vi "UHR-Fleezers Control (host) - Lorentz v2.vi"() -> ()   [LabVIEW 2014] (continued)
                            tunnel: [w3947] -> w3939
                            tunnel: [w3946] -> w3938
                            tunnel: w3937 -> [w3945]
                            tunnel: [w3945] -> w3936
                            tunnel: w3935 -> [w3944]
                            tunnel: [w3944] -> w3934
                            tunnel: [w4020] -> w3942
                            tunnel: w3940 -> [w4020]
                            tunnel: w3939 -> [w4019]
                            tunnel: w3938 -> [w4018]
                            tunnel: w3936 -> [w4017]
                            tunnel: w3934 -> [w4016]
                            frame #0 {
                              n2583 = call <vilib>:"Beep.vi"() -> ()  [unwired: 12 in]
                              n2584 = local write "Waiting"(FALSE ("Waiting")) -> ()
                              n2585 = Increment(x=w3949) -> (x+1=w3948:i32)
                              n2586 = case shown="\"Image\"" w3946 {
                                tunnel: w3948 -> [_ w3954 _]
                                frame "Alarm", Default {
                                }
                                frame "Yank" {
                                n2587 = flat-sequence {
                                tunnel: w3954 -> [w3957]
                                tunnel: [w3956] -> w3953
                                tunnel: [w3955] -> w3952
                                tunnel: w3953 -> [w3967]
                                tunnel: w3952 -> [w3968]
                                frame #0 {
                                n2588 = local read "Yank Delay (s)"() -> (w3960:dbl)
                                n2589 = local read "N Array El"() -> (w3955:u8)
                                n2590 = Quotient & Remainder(x=w3957, y=w3955) -> (x-y*floor(x/y)=w3956:i32)  [unwired: 1 out]
                                n2591 = Multiply(x=w3960, y=1000.0) -> (x*y=w3958:dbl)
                                n2592 = Wait (ms)(milliseconds to wait=w3958) -> ()  [unwired: 1 out]
                                }
                                frame #1 {
                                n2593 = local read "Yank to which?"() -> (w3962:bool)
                                n2594 = local read "Random Choice"() -> (w3972:bool)
                                n2595 = local read "Yank to Trap Delta (MHz)"() -> (w3965:dbl[])
                                n2596 = local read "Yank to SP"() -> (w3966:dbl[])
                                n2597 = Random Number (0-1)() -> (number: 0 to 1=w3971:dbl)
                                n2598 = Multiply(x=w3968, y=w3971) -> (x*y=w3970:dbl)
                                n2599 = Round Toward -Infinity(1:w3970) -> (0:w3969:dbl)
                                n2600 = Select(t=w3969, s=w3972, f=w3967) -> (s? t:f=w3963:dbl)
                                n2601 = Select(t=w3965, s=w3962, f=w3966) -> (s? t:f=w3964:dbl[])
                                n2602 = Index Array(array=w3964, index=w3963) -> (element=w3961:dbl)
                                n2603 = case shown="True" w3962 {
                                tunnel: w3961 -> [w3973 w4000]
                                frame False {
                                n2604 = flat-sequence {
                                tunnel: w3973 -> [w3974]
                                frame #0 {
                                n2605 = property on="Trap Pos FB SP" class="DigNum (strict)"("Val(Sgnl)"=w3974) -> ()  [unwired: 2 in, 2 out]
                                }
                                frame #1 {
                                n2606 = Wait (ms)(milliseconds to wait=u32 700) -> ()  [unwired: 1 out]
                                }
                                frame #2 {
                                n2607 = local read "Action (%)"() -> (w3979:dbl)
                                n2608 = Absolute Value(x=w3979) -> (abs(x)=w3978:dbl)
                                n2609 = Greater?(x=w3978, y=70.0) -> (0:w3976:bool)
                                n2610 = property on="Remove Action Offset" class="Bool (strict)"("Val(Sgnl)"=w3976) -> ()  [unwired: 2 in, 2 out]
                                }
                                frame #3 {
                                n2611 = for {
                                N: 4 -> [_]
                                n2612 = flat-sequence {
                                frame #0 {
                                n2613 = Wait (ms)(milliseconds to wait=u32 500) -> ()  [unwired: 1 out]
                                }
                                frame #1 {
                                n2614 = local read "Action (%)"() -> (w3985:dbl)
                                n2615 = Absolute Value(x=w3985) -> (abs(x)=w3984:dbl)
                                n2616 = Greater?(x=w3984, y=70.0) -> (0:w3982:bool)
                                n2617 = property on="Remove Action Offset" class="Bool (strict)"("Val(Sgnl)"=w3982) -> ()  [unwired: 2 in, 2 out]
                                }
                                }
                                }
                                }
                                frame #4 {
                                n2618 = Wait (ms)(milliseconds to wait=u32 500) -> ()  [unwired: 1 out]
                                }
                                frame #5 {
                                n2619 = local read "Mean"() -> (w3993:dbl)
                                n2620 = Greater?(x=w3993, y=11.0) -> (0:w3987:bool)
                                n2621 = Not(x=w3987) -> (.not. x?=w3988:bool)
                                n2622 = And(x=w3988, y="Shift confocal") -> (x .and. y?=w3990:bool)
                                n2623 = And(x=w3987, y="Shift confocal") -> (x .and. y?=w3991:bool)
                                n2624 = case shown="True" w3991 {
                                frame False {
                                }
                                frame True {
                                n2625 = local read "Confocal Y 2 (V)"() -> (w3997:dbl)
                                n2626 = local read "Confocal X 2 (V)"() -> (w3996:dbl)
                                n2627 = property on="AO1" class="Slide (strict)"("Val(Sgnl)"=w3997) -> ()  [unwired: 2 in, 2 out]
                                n2628 = property on="AO2" class="Slide (strict)"("Val(Sgnl)"=w3996) -> ()  [unwired: 2 in, 2 out]
                                }
                                }
                                n2629 = case shown="True" w3990 {
                                frame False {
                                }
                                frame True {
                                n2630 = local read "Confocal Y 1 (V)"() -> (w3995:dbl)
                                n2631 = local read "Confocal X 1 (V)"() -> (w3994:dbl)
                                n2632 = property on="AO1" class="Slide (strict)"("Val(Sgnl)"=w3995) -> ()  [unwired: 2 in, 2 out]
                                n2633 = property on="AO2" class="Slide (strict)"("Val(Sgnl)"=w3994) -> ()  [unwired: 2 in, 2 out]
                                }
                                }
                                }
                                frame #6 {
                                n2634 = Wait (ms)(milliseconds to wait=u32 1500) -> ()  [unwired: 1 out]
                                }
                                frame #7 {
                                n2635 = property on="Rem fb disp offset" class="Bool (strict)"("Val(Sgnl)"=TRUE ("Value (Signaling)")) -> ()  [unwired: 2 in, 2 out]
                                }
                                }
                                }
                                frame True {
                                n2636 = flat-sequence {
                                tunnel: w4000 -> [w4001]
                                frame #0 {
                                n2637 = property on="Trap Delta (MHz)" class="DigNum (strict)"("Val(Sgnl)"=w4001) -> ()  [unwired: 2 in, 2 out]
                                }
                                frame #1 {
                                n2638 = Wait (ms)(milliseconds to wait=u32 500) -> ()  [unwired: 1 out]
                                }
                                frame #2 {
                                n2639 = local read "Shift confocal"() -> (w4007:bool)
                                n2640 = local read "Mean"() -> (w4009:dbl)
                                n2641 = Greater?(x=w4009, y=11.0) -> (0:w4006:bool)
                                n2642 = Not(x=w4006) -> (.not. x?=w4005:bool)
                                n2643 = And(x=w4005, y=w4007) -> (x .and. y?=w4003:bool)
                                n2644 = And(x=w4006, y=w4007) -> (x .and. y?=w4004:bool)
                                n2645 = case shown="True" w4004 {
                                frame False {
                                }
                                frame True {
                                n2646 = local read "Confocal Y 2 (V)"() -> (w4013:dbl)
                                n2647 = local read "Confocal X 2 (V)"() -> (w4012:dbl)
                                n2648 = property on="AO2" class="Slide (strict)"("Val(Sgnl)"=w4012) -> ()  [unwired: 2 in, 2 out]
                                n2649 = property on="AO1" class="Slide (strict)"("Val(Sgnl)"=w4013) -> ()  [unwired: 2 in, 2 out]
                                }
                                }
                                n2650 = case shown="True" w4003 {
                                frame False {
                                }
                                frame True {
                                n2651 = local read "Confocal X 1 (V)"() -> (w4010:dbl)
                                n2652 = local read "Confocal Y 1 (V)"() -> (w4011:dbl)
                                n2653 = property on="AO2" class="Slide (strict)"("Val(Sgnl)"=w4010) -> ()  [unwired: 2 in, 2 out]
                                n2654 = property on="AO1" class="Slide (strict)"("Val(Sgnl)"=w4011) -> ()  [unwired: 2 in, 2 out]
                                }
                                }
                                }
                                }
                                }
                                }
                                }
                                }
                                }
                                frame "Image" {
                                n2655 = property on="Confocal Image" class="Bool (strict)"("Val(Sgnl)"=TRUE ("Value (Signaling)")) -> ()  [unwired: 2 in, 2 out]
                                }
                              }
                              n2656 = local write "Fl. High"(FALSE ("Fl. High")) -> ()
                              n2657 = local read "Time (s)"() -> (w3947:dbl)
                            }
                            frame #1 {
                              n2658 = case shown="True" "Auto F Reset" {
                                tunnel: w4019 -> [_ w4024]
                                tunnel: w4018 -> [_ w4023]
                                tunnel: w4017 -> [_ w4022]
                                tunnel: w4016 -> [_ w4021]
                                frame False {
                                }
                                frame True {
                                n2659 = node-c288() -> (w4026:T35)  [unwired: 4 in]
                                n2660 = timed-loop {
                                timing: w4026 -> [_]
                                timing-out: [_] -> w4025
                                tunnel: w4024 -> [w4031]
                                tunnel: w4023 -> [w4030]
                                tunnel: w4022 -> [w4029]
                                tunnel: w4021 -> [w4028]
                                stop <- w4027 stop-if-true
                                n2661 = node-c288() -> ()  [unwired: 1 in, 1 out]
                                n2662 = local read "Fl. Delta Thresh. (kHz)"() -> (w4040:dbl)
                                n2663 = local read "APD to Watch"() -> (w4041:bool)
                                n2664 = local read "Delta Fl. 1"() -> (w4042:dbl)
                                n2665 = local read "Delta Fl. 2"() -> (w4043:dbl)
                                n2666 = local read "Fl. Triggered..."() -> (w4034:bool)
                                n2667 = local read "Stop All"() -> (w4035:bool)
                                n2668 = local read "Reset Force"() -> (w4033:bool)
                                n2669 = Multiply(x=w4040, y=1000.0) -> (x*y=w4038:dbl)
                                n2670 = Select(t=w4042, s=w4041, f=w4043) -> (s? t:f=w4037:dbl)
                                n2671 = Not(x=w4034) -> (.not. x?=w4032:bool)
                                n2672 = Greater?(x=w4037, y=w4038) -> (0:w4036:bool)
                                n2673 = Compound Arithmetic op=OR(w4036, w4035, w4032, w4033) -> (w4027:bool)
                                n2674 = case shown="True" w4027 {
                                tunnel: w4031 -> [_ w4047]
                                tunnel: w4030 -> [_ w4051]
                                tunnel: w4029 -> [_ w4050]
                                tunnel: w4028 -> [_ w4049]
                                frame False {
                                }
                                frame True {
                                n2675 = case shown="\"Yank\"" w4051 {
                                tunnel: w4050 -> [_ w4061]
                                tunnel: w4049 -> [_ w4059]
                                frame "Image", Default {
                                }
                                frame "Yank" {
                                n2676 = flat-sequence {
                                tunnel: [w4064] -> w4062
                                tunnel: w4061 -> [w4064]
                                tunnel: [w4063] -> w4060
                                tunnel: w4059 -> [w4063]
                                tunnel: w4062 -> [w4070]
                                tunnel: w4060 -> [w4068]
                                frame #0 {
                                n2677 = local read "Yank Delay (s)"() -> (w4067:dbl)
                                n2678 = Multiply(x=w4067, y=1000.0) -> (x*y=w4065:dbl)
                                n2679 = Wait (ms)(milliseconds to wait=w4065) -> ()  [unwired: 1 out]
                                }
                                frame #1 {
                                n2680 = local read "Yank to which?"() -> (w4069:bool)
                                n2681 = case shown="False" w4069 {
                                tunnel: w4070 -> [_ w4098]
                                tunnel: w4068 -> [w4071 _]
                                frame False {
                                n2682 = flat-sequence {
                                tunnel: w4071 -> [w4072]
                                frame #0 {
                                n2683 = property on="Trap Pos FB SP" class="DigNum (strict)"("Val(Sgnl)"=w4072) -> ()  [unwired: 2 in, 2 out]
                                }
                                frame #1 {
                                n2684 = Wait (ms)(milliseconds to wait=u32 700) -> ()  [unwired: 1 out]
                                }
                                frame #2 {
                                n2685 = local read "Action (%)"() -> (w4077:dbl)
                                n2686 = Absolute Value(x=w4077) -> (abs(x)=w4076:dbl)
                                n2687 = Greater?(x=w4076, y=70.0) -> (0:w4074:bool)
                                n2688 = property on="Remove Action Offset" class="Bool (strict)"("Val(Sgnl)"=w4074) -> ()  [unwired: 2 in, 2 out]
                                }
                                frame #3 {
                                n2689 = for {
                                N: 4 -> [_]
                                n2690 = flat-sequence {
                                frame #0 {
                                n2691 = Wait (ms)(milliseconds to wait=u32 500) -> ()  [unwired: 1 out]
                                }
                                frame #1 {
                                n2692 = local read "Action (%)"() -> (w4083:dbl)
                                n2693 = Absolute Value(x=w4083) -> (abs(x)=w4082:dbl)
                                n2694 = Greater?(x=w4082, y=70.0) -> (0:w4080:bool)
                                n2695 = property on="Remove Action Offset" class="Bool (strict)"("Val(Sgnl)"=w4080) -> ()  [unwired: 2 in, 2 out]
                                }
                                }
                                }
                                }
                                frame #4 {
                                n2696 = Wait (ms)(milliseconds to wait=u32 500) -> ()  [unwired: 1 out]
                                }
                                frame #5 {
                                n2697 = local read "Shift confocal"() -> (w4088:bool)
                                n2698 = local read "Mean"() -> (w4091:dbl)
                                n2699 = Greater?(x=w4091, y=11.0) -> (0:w4087:bool)
                                n2700 = Not(x=w4087) -> (.not. x?=w4086:bool)
                                n2701 = And(x=w4087, y=w4088) -> (x .and. y?=w4089:bool)
                                n2702 = And(x=w4086, y=w4088) -> (x .and. y?=w4085:bool)
                                n2703 = case shown="True" w4089 {
                                frame False {
                                }
                                frame True {
                                n2704 = local read "Confocal X 2 (V)"() -> (w4094:dbl)
                                n2705 = local read "Confocal Y 2 (V)"() -> (w4095:dbl)
                                n2706 = property on="AO2" class="Slide (strict)"("Val(Sgnl)"=w4094) -> ()  [unwired: 2 in, 2 out]
                                n2707 = property on="AO1" class="Slide (strict)"("Val(Sgnl)"=w4095) -> ()  [unwired: 2 in, 2 out]
                                }
                                }
                                n2708 = case shown="True" w4085 {
                                frame False {
                                }
                                frame True {
                                n2709 = local read "Confocal Y 1 (V)"() -> (w4093:dbl)
                                n2710 = local read "Confocal X 1 (V)"() -> (w4092:dbl)
                                n2711 = property on="AO1" class="Slide (strict)"("Val(Sgnl)"=w4093) -> ()  [unwired: 2 in, 2 out]
                                n2712 = property on="AO2" class="Slide (strict)"("Val(Sgnl)"=w4092) -> ()  [unwired: 2 in, 2 out]
                                }
                                }
                                }
                                frame #6 {
                                n2713 = Wait (ms)(milliseconds to wait=u32 1500) -> ()  [unwired: 1 out]
                                }
                                frame #7 {
                                n2714 = property on="Rem fb disp offset" class="Bool (strict)"("Val(Sgnl)"=TRUE ("Value (Signaling)")) -> ()  [unwired: 2 in, 2 out]
                                }
                                }
                                }
                                frame True {
                                n2715 = flat-sequence {
                                tunnel: w4098 -> [w4099]
                                frame #0 {
                                n2716 = property on="Trap Delta (MHz)" class="DigNum (strict)"("Val(Sgnl)"=w4099) -> ()  [unwired: 2 in, 2 out]
                                }
                                frame #1 {
                                n2717 = Wait (ms)(milliseconds to wait=u32 500) -> ()  [unwired: 1 out]
                                }
                                frame #2 {
                                n2718 = local read "Shift confocal"() -> (w4105:bool)
                                n2719 = local read "Mean"() -> (w4106:dbl)
                                n2720 = Greater?(x=w4106, y=11.0) -> (0:w4104:bool)
                                n2721 = And(x=w4104, y=w4105) -> (x .and. y?=w4102:bool)
                                n2722 = Not(x=w4104) -> (.not. x?=w4103:bool)
                                n2723 = And(x=w4103, y=w4105) -> (x .and. y?=w4101:bool)
                                n2724 = case shown="True" w4102 {
                                frame False {
                                }
                                frame True {
                                n2725 = local read "Confocal Y 2 (V)"() -> (w4111:dbl)
                                n2726 = local read "Confocal X 2 (V)"() -> (w4110:dbl)
                                n2727 = property on="AO1" class="Slide (strict)"("Val(Sgnl)"=w4111) -> ()  [unwired: 2 in, 2 out]
                                n2728 = property on="AO2" class="Slide (strict)"("Val(Sgnl)"=w4110) -> ()  [unwired: 2 in, 2 out]
                                }
                                }
                                n2729 = case shown="True" w4101 {
                                frame False {
                                }
                                frame True {
                                n2730 = local read "Confocal Y 1 (V)"() -> (w4109:dbl)
                                n2731 = local read "Confocal X 1 (V)"() -> (w4108:dbl)
                                n2732 = property on="AO2" class="Slide (strict)"("Val(Sgnl)"=w4108) -> ()  [unwired: 2 in, 2 out]
                                n2733 = property on="AO1" class="Slide (strict)"("Val(Sgnl)"=w4109) -> ()  [unwired: 2 in, 2 out]
                                }
                                }
                                }
                                }
                                }
                                }
                                }
                                }
                                }
                                }
                                n2734 = local read "Time (s)"() -> (w4046:dbl)
                                n2735 = Subtract(x=w4047, y=w4046) -> (x-y=w4058:dbl)
                                n2736 = Number To Decimal String(number=w4058, width (-)=i16 0) -> (decimal integer string=w4056:string)
                                n2737 = Concatenate Strings(w4056, " s fluorescence event") -> (w4053:string)
                                n2738 = local read "Messages"() -> (w4054:string)
                                n2739 = local write "Duration (s)"(w4058) -> ()
                                n2740 = call "Update messages.vi"("Message to add"=w4053, "Old message string"=w4054) -> ("New message string"=w4052:string)
                                n2741 = local write "Messages"(w4052) -> ()
                                n2742 = call <vilib>:"Beep.vi"() -> ()  [unwired: 12 in]
                                n2743 = local write "Reset Force"(FALSE ("Force Reset")) -> ()
                                n2744 = local write "Fl. High"(TRUE ("Fl. High")) -> ()
                                n2745 = local write "Waiting"(TRUE ("Waiting")) -> ()
                                }
                                }
                                n2746 = node-c288() -> ()  [unwired: 1 in, 1 out]
                                }
                                n2747 = node-c288(w4025) -> ()  [unwired: 1 out]
                                }
                              }
                            }
                          }
                          n2748 = local read "Trap Delta (MHz)"() -> (w3937:dbl)
                          n2749 = local read "Trap Pos FB SP"() -> (w3935:fxp<+/-,16,1>)
                        }
                      }
                    }
                    frame True {
                      n2750 = flat-sequence {
                        tunnel: w4122 -> [w4132]
                        tunnel: [w4132] -> w4126
                        tunnel: w4125 -> [w4131]
                        tunnel: [w4131] -> w4124
                        tunnel: [w4130] -> w4123
                        tunnel: w4121 -> [w4129]
                        tunnel: [w4128] -> w4120
                        tunnel: w4117 -> [w4127]
                        tunnel: [w4127] -> w4116
                        tunnel: w4126 -> [w4202]
                        tunnel: w4124 -> [w4201]
                        tunnel: w4123 -> [w4200]
                        tunnel: w4120 -> [w4199]
                        tunnel: w4116 -> [w4198]
                        tunnel: [w4199] -> w4119
                        frame #0 {
                          n2751 = call <vilib>:"Beep.vi"() -> ()  [unwired: 3 in, 9 out]
                          n2752 = local write "Waiting"(FALSE ("Waiting")) -> ()
                          n2753 = Increment(x=w4129) -> (x+1=w4128:u8)
                          n2754 = case shown="\"Image\"" w4131 {
                            tunnel: w4128 -> [_ _ w4138]
                            frame "Image" {
                              n2755 = property on="Confocal Image" class="Bool (strict)"("Val(Sgnl)"=TRUE ("Value (Signaling)")) -> ()  [unwired: 2 in, 2 out]
                            }
                            frame "Alarm", Default {
                            }
                            frame "Yank" {
                              n2756 = flat-sequence {
                                tunnel: w4138 -> [w4141]
                                tunnel: [w4140] -> w4137
                                tunnel: ["N Array El"] -> w4136
                                tunnel: w4137 -> [w4155]
                                tunnel: w4136 -> [w4151]
                                frame #0 {
                                n2757 = Multiply(x="Yank Delay (s)", y=1000.0) -> (x*y=w4144:dbl)
                                n2758 = Quotient & Remainder(x=w4141, y="N Array El") -> (x-y*floor(x/y)=w4140:u8)  [unwired: 1 out]
                                n2759 = Wait (ms)(milliseconds to wait=w4144) -> ()  [unwired: 1 out]
                                }
                                frame #1 {
                                n2760 = Random Number (0-1)() -> (number: 0 to 1=w4152:dbl)
                                n2761 = Multiply(x=w4151, y=w4152) -> (x*y=w4150:dbl)
                                n2762 = Round Toward -Infinity(1:w4150) -> (0:w4149:dbl)
                                n2763 = Select(t=w4149, s="Random Choice", f=w4155) -> (s? t:f=w4153:dbl)
                                n2764 = Select(t="Yank to Trap Delta (MHz)", s="Yank to which?", f="Yank to SP") -> (s? t:f=w4146:dbl[])
                                n2765 = Index Array(array=w4146, index=w4153) -> (element=w4156:dbl)
                                n2766 = case shown="False" "Yank to which?" {
                                tunnel: w4156 -> [w4157 w4183]
                                frame False {
                                n2767 = flat-sequence {
                                tunnel: w4157 -> [w4158]
                                frame #0 {
                                n2768 = property on="Trap Pos FB SP" class="DigNum (strict)"("Val(Sgnl)"=w4158) -> ()  [unwired: 2 in, 2 out]
                                }
                                frame #1 {
                                n2769 = Wait (ms)(milliseconds to wait=u32 700) -> ()  [unwired: 1 out]
                                }
                                frame #2 {
                                n2770 = local read "Action (%)"() -> (w4163:dbl)
                                n2771 = Absolute Value(x=w4163) -> (abs(x)=w4162:dbl)
                                n2772 = Greater?(x=w4162, y=70.0) -> (0:w4160:bool)
                                n2773 = property on="Remove Action Offset" class="Bool (strict)"("Val(Sgnl)"=w4160) -> ()  [unwired: 2 in, 2 out]
                                }
                                frame #3 {
                                n2774 = for {
                                N: 4 -> [_]
                                n2775 = flat-sequence {
                                frame #0 {
                                n2776 = Wait (ms)(milliseconds to wait=u32 500) -> ()  [unwired: 1 out]
                                }
                                frame #1 {
                                n2777 = local read "Action (%)"() -> (w4169:dbl)
                                n2778 = Absolute Value(x=w4169) -> (abs(x)=w4168:dbl)
                                n2779 = Greater?(x=w4168, y=70.0) -> (0:w4166:bool)
                                n2780 = property on="Remove Action Offset" class="Bool (strict)"("Val(Sgnl)"=w4166) -> ()  [unwired: 2 in, 2 out]
                                }
                                }
                                }
                                }
                                frame #4 {
                                n2781 = local read "Shift confocal"() -> (w4173:bool)
                                n2782 = local read "Mean"() -> (w4176:dbl)
                                n2783 = Greater?(x=w4176, y=11.0) -> (0:w4172:bool)
                                n2784 = Not(x=w4172) -> (.not. x?=w4171:bool)
                                n2785 = And(x=w4171, y=w4173) -> (x .and. y?=w4170:bool)
                                n2786 = And(x=w4172, y=w4173) -> (x .and. y?=w4174:bool)
                                n2787 = case shown="True" w4174 {
                                frame False {
                                }
                                frame True {
                                n2788 = local read "Confocal X 2 (V)"() -> (w4179:dbl)
                                n2789 = local read "Confocal Y 2 (V)"() -> (w4180:dbl)
                                n2790 = property on="AO2" class="Slide (strict)"("Val(Sgnl)"=w4179) -> ()  [unwired: 2 in, 2 out]
                                n2791 = property on="AO1" class="Slide (strict)"("Val(Sgnl)"=w4180) -> ()  [unwired: 2 in, 2 out]
                                }
                                }
                                n2792 = case shown="True" w4170 {
                                frame False {
                                }
                                frame True {
                                n2793 = local read "Confocal X 1 (V)"() -> (w4177:dbl)
                                n2794 = local read "Confocal Y 1 (V)"() -> (w4178:dbl)
                                n2795 = property on="AO1" class="Slide (strict)"("Val(Sgnl)"=w4178) -> ()  [unwired: 2 in, 2 out]
                                n2796 = property on="AO2" class="Slide (strict)"("Val(Sgnl)"=w4177) -> ()  [unwired: 2 in, 2 out]
                                }
                                }
                                }
                                frame #5 {
                                n2797 = Wait (ms)(milliseconds to wait=u32 1500) -> ()  [unwired: 1 out]
                                }
                                frame #6 {
                                n2798 = property on="Rem fb disp offset" class="Bool (strict)"("Val(Sgnl)"=TRUE ("Value (Signaling)")) -> ()  [unwired: 2 in, 2 out]
                                }
                                }
                                }
                                frame True {
                                n2799 = flat-sequence {
                                tunnel: w4183 -> [w4184]
                                frame #0 {
                                n2800 = property on="Trap Delta (MHz)" class="DigNum (strict)"("Val(Sgnl)"=w4184) -> ()  [unwired: 2 in, 2 out]
                                }
                                frame #1 {
                                n2801 = Wait (ms)(milliseconds to wait=u32 500) -> ()  [unwired: 1 out]
                                }
                                frame #2 {
                                n2802 = local read "Shift confocal"() -> (w4188:bool)
                                n2803 = local read "Mean"() -> (w4186:dbl)
                                n2804 = Greater?(x=w4186, y=11.0) -> (0:w4189:bool)
                                n2805 = Not(x=w4189) -> (.not. x?=w4190:bool)
                                n2806 = And(x=w4190, y=w4188) -> (x .and. y?=w4192:bool)
                                n2807 = And(x=w4189, y=w4188) -> (x .and. y?=w4191:bool)
                                n2808 = case shown="True" w4191 {
                                frame False {
                                }
                                frame True {
                                n2809 = local read "Confocal Y 2 (V)"() -> (w4196:dbl)
                                n2810 = local read "Confocal X 2 (V)"() -> (w4195:dbl)
                                n2811 = property on="AO1" class="Slide (strict)"("Val(Sgnl)"=w4196) -> ()  [unwired: 2 in, 2 out]
                                n2812 = property on="AO2" class="Slide (strict)"("Val(Sgnl)"=w4195) -> ()  [unwired: 2 in, 2 out]
                                }
                                }
                                n2813 = case shown="True" w4192 {
                                frame False {
                                }
                                frame True {
                                n2814 = local read "Confocal X 1 (V)"() -> (w4193:dbl)
                                n2815 = local read "Confocal Y 1 (V)"() -> (w4194:dbl)
                                n2816 = property on="AO2" class="Slide (strict)"("Val(Sgnl)"=w4193) -> ()  [unwired: 2 in, 2 out]
                                n2817 = property on="AO1" class="Slide (strict)"("Val(Sgnl)"=w4194) -> ()  [unwired: 2 in, 2 out]
                                }
                                }
                                }
                                }
                                }
                                }
                                }
                              }
                            }
                          }
                          n2818 = local read "Time (s)"() -> (w4130:dbl)
                          "Fl. High" <- TRUE ("Yanking")
                        }
                        frame #1 {
                          n2819 = local read "Auto F Reset"() -> (w4197:bool)
                          n2820 = case shown="True" w4197 {
                            tunnel: w4202 -> [_ w4206]
                            tunnel: w4201 -> [_ w4205]
                            tunnel: w4200 -> [_ w4204]
                            tunnel: w4198 -> [_ w4203]
                            frame False {
                            }
                            frame True {
                              n2821 = node-c288() -> (w4208:T35)  [unwired: 4 out]
                              n2822 = timed-loop {
                                timing: w4208 -> [_]
                                timing-out: [_] -> w4207
                                tunnel: w4206 -> [w4226]
                                tunnel: w4205 -> [w4225]
                                tunnel: w4204 -> [w4224]
                                tunnel: w4203 -> [w4223]
                                stop <- w4209 stop-if-true
                                n2823 = node-c288() -> ()  [unwired: 2 out]
                                n2824 = local read "Fl. Delta Thresh. (kHz)"() -> (w4217:dbl)
                                n2825 = local read "Fl. Triggered..."() -> (w4222:bool)
                                n2826 = local read "Delta Fl. 1"() -> (w4213:dbl)
                                n2827 = local read "Delta Fl. 2"() -> (w4211:dbl)
                                n2828 = local read "Stop All"() -> (w4220:bool)
                                n2829 = local read "APD to Watch"() -> (w4212:bool)
                                n2830 = Select(t=w4213, s=w4212, f=w4211) -> (s? t:f=w4210:dbl)
                                n2831 = Not(x=w4222) -> (.not. x?=w4221:bool)
                                n2832 = Multiply(x=w4217, y=1000.0) -> (x*y=w4216:dbl)
                                n2833 = Negate(x=w4216) -> (-x=w4215:dbl)
                                n2834 = Less?(x=w4210, y=w4215) -> (x < y?=w4219:bool)
                                n2835 = Compound Arithmetic op=OR(w4219, w4220, w4221, "Reset Force") -> (w4209:bool)
                                n2836 = case shown="True" w4209 {
                                tunnel: w4226 -> [_ w4241]
                                tunnel: w4225 -> [_ w4240]
                                tunnel: w4224 -> [_ w4230]
                                tunnel: w4223 -> [_ w4232]
                                frame False {
                                }
                                frame True {
                                n2837 = local read "Time (s)"() -> (w4231:dbl)
                                n2838 = case shown="\"Yank\"" w4240 {
                                tunnel: w4241 -> [_ w4244]
                                tunnel: w4232 -> [_ w4242]
                                frame "Image", Default {
                                }
                                frame "Yank" {
                                n2839 = flat-sequence {
                                tunnel: [w4250] -> w4245
                                tunnel: w4244 -> [w4250]
                                tunnel: [w4246] -> w4243
                                tunnel: w4242 -> [w4246]
                                tunnel: w4245 -> [w4253]
                                tunnel: w4243 -> [w4251]
                                frame #0 {
                                n2840 = local read "Yank Delay (s)"() -> (w4249:dbl)
                                n2841 = Multiply(x=w4249, y=1000.0) -> (x*y=w4247:dbl)
                                n2842 = Wait (ms)(milliseconds to wait=w4247) -> ()  [unwired: 1 out]
                                }
                                frame #1 {
                                n2843 = local read "Yank to which?"() -> (w4252:bool)
                                n2844 = case shown="False" w4252 {
                                tunnel: w4253 -> [_ w4280]
                                tunnel: w4251 -> [w4254 _]
                                frame False {
                                n2845 = flat-sequence {
                                tunnel: w4254 -> [w4255]
                                frame #0 {
                                n2846 = property on="Trap Pos FB SP" class="DigNum (strict)"("Val(Sgnl)"=w4255) -> ()  [unwired: 2 in, 2 out]
                                }
                                frame #1 {
                                n2847 = Wait (ms)(milliseconds to wait=u32 700) -> ()  [unwired: 1 out]
                                }
                                frame #2 {
                                n2848 = local read "Action (%)"() -> (w4260:dbl)
                                n2849 = Absolute Value(x=w4260) -> (abs(x)=w4259:dbl)
                                n2850 = Greater?(x=w4259, y=70.0) -> (0:w4257:bool)
                                n2851 = property on="Remove Action Offset" class="Bool (strict)"("Val(Sgnl)"=w4257) -> ()  [unwired: 2 in, 2 out]
                                }
                                frame #3 {
                                n2852 = for {
                                N: 4 -> [_]
                                n2853 = flat-sequence {
                                frame #0 {
                                n2854 = Wait (ms)(milliseconds to wait=u32 500) -> ()  [unwired: 1 out]
                                }
                                frame #1 {
                                n2855 = local read "Action (%)"() -> (w4266:dbl)
                                n2856 = Absolute Value(x=w4266) -> (abs(x)=w4265:dbl)
                                n2857 = Greater?(x=w4265, y=70.0) -> (0:w4263:bool)
                                n2858 = property on="Remove Action Offset" class="Bool (strict)"("Val(Sgnl)"=w4263) -> ()  [unwired: 2 in, 2 out]
                                }
                                }
                                }
                                }
                                frame #4 {
                                n2859 = local read "Shift confocal"() -> (w4271:bool)
                                n2860 = local read "Mean"() -> (w4273:dbl)
                                n2861 = Greater?(x=w4273, y=11.0) -> (0:w4270:bool)
                                n2862 = Not(x=w4270) -> (.not. x?=w4269:bool)
                                n2863 = And(x=w4270, y=w4271) -> (x .and. y?=w4268:bool)
                                n2864 = And(x=w4269, y=w4271) -> (x .and. y?=w4267:bool)
                                n2865 = case shown="True" w4268 {
                                frame False {
                                }
                                frame True {
                                n2866 = local read "Confocal Y 2 (V)"() -> (w4277:dbl)
                                n2867 = local read "Confocal X 2 (V)"() -> (w4276:dbl)
                                n2868 = property on="AO2" class="Slide (strict)"("Val(Sgnl)"=w4276) -> ()  [unwired: 2 in, 2 out]
                                n2869 = property on="AO1" class="Slide (strict)"("Val(Sgnl)"=w4277) -> ()  [unwired: 2 in, 2 out]
                                }
                                }
                                n2870 = case shown="True" w4267 {
                                frame False {
                                }
                                frame True {
                                n2871 = local read "Confocal X 1 (V)"() -> (w4274:dbl)
                                n2872 = local read "Confocal Y 1 (V)"() -> (w4275:dbl)
                                n2873 = property on="AO1" class="Slide (strict)"("Val(Sgnl)"=w4275) -> ()  [unwired: 2 in, 2 out]
                                n2874 = property on="AO2" class="Slide (strict)"("Val(Sgnl)"=w4274) -> ()  [unwired: 2 in, 2 out]
                                }
                                }
                                }
                                frame #5 {
                                n2875 = Wait (ms)(milliseconds to wait=u32 1500) -> ()  [unwired: 1 out]
                                }
                                frame #6 {
                                n2876 = property on="Rem fb disp offset" class="Bool (strict)"("Val(Sgnl)"=TRUE ("Value (Signaling)")) -> ()  [unwired: 2 in, 2 out]
                                }
                                }
                                }
                                frame True {
                                n2877 = flat-sequence {
                                tunnel: w4280 -> [w4281]
                                frame #0 {
                                n2878 = property on="Trap Delta (MHz)" class="DigNum (strict)"("Val(Sgnl)"=w4281) -> ()  [unwired: 2 in, 2 out]
                                }
                                frame #1 {
                                n2879 = Wait (ms)(milliseconds to wait=u32 500) -> ()  [unwired: 1 out]
                                }
                                frame #2 {
                                n2880 = local read "Shift confocal"() -> (w4287:bool)
                                n2881 = local read "Mean"() -> (w4289:dbl)
                                n2882 = Greater?(x=w4289, y=11.0) -> (0:w4286:bool)
                                n2883 = Not(x=w4286) -> (.not. x?=w4285:bool)
                                n2884 = And(x=w4286, y=w4287) -> (x .and. y?=w4284:bool)
                                n2885 = And(x=w4285, y=w4287) -> (x .and. y?=w4283:bool)
                                n2886 = case shown="True" w4284 {
                                frame False {
                                }
                                frame True {
                                n2887 = local read "Confocal Y 2 (V)"() -> (w4293:dbl)
                                n2888 = local read "Confocal X 2 (V)"() -> (w4292:dbl)
                                n2889 = property on="AO2" class="Slide (strict)"("Val(Sgnl)"=w4292) -> ()  [unwired: 2 in, 2 out]
                                n2890 = property on="AO1" class="Slide (strict)"("Val(Sgnl)"=w4293) -> ()  [unwired: 2 in, 2 out]
                                }
                                }
                                n2891 = case shown="True" w4283 {
                                frame False {
                                }
                                frame True {
                                n2892 = local read "Confocal Y 1 (V)"() -> (w4291:dbl)
                                n2893 = local read "Confocal X 1 (V)"() -> (w4290:dbl)
                                n2894 = property on="AO2" class="Slide (strict)"("Val(Sgnl)"=w4290) -> ()  [unwired: 2 in, 2 out]
                                n2895 = property on="AO1" class="Slide (strict)"("Val(Sgnl)"=w4291) -> ()  [unwired: 2 in, 2 out]
                                }
                                }
                                }
                                }
                                }
                                }
                                }
                                }
                                }
                                }
                                n2896 = local read "Messages"() -> (w4239:string)
                                n2897 = Subtract(x=w4231, y=w4230) -> (x-y=w4237:dbl)
                                "Duration (s)" <- w4237
                                n2898 = Number To Decimal String(number=w4237, width (-)=i16 0) -> (decimal integer string=w4235:string)
                                n2899 = Concatenate Strings(w4235, " s fluorescence event." ("string")) -> (w4233:string)
                                n2900 = call "Update messages.vi"("Message to add"=w4233, "Old message string"=w4239) -> ("New message string"=w4238:string)
                                n2901 = local write "Reset Force"(FALSE ("Reset Force")) -> ()
                                n2902 = local write "Waiting"(TRUE ("Waiting")) -> ()
                                n2903 = local write "Messages"(w4238) -> ()
                                n2904 = local write "Fl. High"(FALSE ("Fl. High")) -> ()
                                n2905 = call <vilib>:"Beep.vi"() -> ()  [unwired: 3 in, 9 out]
                                }
                                }
                                n2906 = node-c288() -> ()  [unwired: 2 out]
                              }
                              n2907 = node-c288(w4207) -> ()  [unwired: 1 out]
                            }
                          }
                        }
                      }
                      n2908 = local read "Trap Delta (MHz)"() -> (w4122:dbl)
                      n2909 = local read "Trap Pos FB SP"() -> (w4117:fxp<+/-,16,1>)
                    }
                  }
                }
                frame #1 {
                  n2910 = local read "Stop All"() -> (w4303:bool)
                  n2911 = local read "Fl. Triggered..."() -> (w4301:bool)
                  n2912 = Not(x=w4301) -> (.not. x?=w4302:bool)
                  n2913 = Or(x=w4302, y=w4303) -> (x .or. y?=w4300:bool)
                }
              }
              n2914 = case shown="True" w3894 {
                frame False {
                }
                frame True {
                  n2915 = local read "Confocal Y 1 (V)"() -> (w3904:dbl)
                  n2916 = local read "Confocal X 1 (V)"() -> (w3903:dbl)
                  n2917 = property on="AO2" class="Slide (strict)"("Val(Sgnl)"=w3903) -> ()  [unwired: 2 in, 2 out]
                  n2918 = property on="AO1" class="Slide (strict)"("Val(Sgnl)"=w3904) -> ()  [unwired: 2 in, 2 out]
                }
              }
              n2919 = case shown="True" w3894 {
                frame False {
                }
                frame True {
                  w3902 = FALSE ("Fl. High")
                  n2920 = local write "Waiting"(w3902) -> ()
                  n2921 = local write "Fl. High"(w3902) -> ()
                }
              }
              n2922 = node-c288() -> ()  [unwired: 2 out]
            }
            n2923 = node-c288(w3892) -> ()  [unwired: 1 out]
          }
        }
      }
      event "Start assembly line": Value Change {
        n2924 = event-data() -> ()  [unwired: 7 out]
        n2925 = case shown="True" "Start assembly line" {
          tunnel: w4309 -> [_ w4310]
          frame False {
          }
          frame True {
            n2926 = flat-sequence {
              tunnel: w4310 -> [w4315]
              tunnel: [w4314] -> w4312
              tunnel: w4312 -> [w4346]
              tunnel: [w4345] -> w4311
              tunnel: w4311 -> [w4348]
              tunnel: w4310 -> [w4366]
              frame #0 {
                w4313 = TRUE ("Value (Signaling)")
                n2927 = property on="Green Laser ON" class="Bool (strict)"("Val(Sgnl)"=w4313) -> ()  [unwired: 2 in, 2 out]
                "AL Running" <- w4313
              }
              frame #1 {
                n2928 = node-c288() -> (w4317:T35)  [unwired: 4 in]
                n2929 = timed-loop {
                  timing: w4317 -> [_]
                  timing-out: [_] -> w4316
                  tunnel: w4315 -> [w4324]
                  tunnel: [w4318] -> w4314
                  stop <- w4320 stop-if-true
                  n2930 = node-c288() -> ()  [unwired: 1 in, 1 out]
                  n2931 = local read "APD 1 Rate (Hz)"() -> (w4319:dbl)
                  n2932 = Multiply(x="Cy3 Fl.  Thresh. (kHz)", y=1000.0) -> (x*y=w4327:dbl)
                  n2933 = Greater?(x=w4319, y=w4327) -> (0:w4323:bool)
                  n2934 = case shown="True" w4323 {
                    tunnel: w4324 -> [_ w4330]
                    tunnel: [TRUE ("Stage Moving") w4329] -> w4322
                    frame False {
                    }
                    frame True {
                      n2935 = flat-sequence {
                        tunnel: w4330 -> [w4335]
                        tunnel: [w4340] -> w4329
                        frame #0 {
                          n2936 = Multiply(x="AL Delay (s)", y=u32 1000) -> (x*y=w4332:u32)
                          n2937 = Wait (ms)(milliseconds to wait=w4332) -> ()  [unwired: 1 out]
                        }
                        frame #1 {
                          n2938 = property on="Green Laser ON" class="Bool (strict)"("Val(Sgnl)"=FALSE ("Value (Signaling)")) -> ()  [unwired: 2 in, 2 out]
                        }
                        frame #2 {
                          # "upper spot"
                          n2939 = local read "Saved Stage Positions"() -> (w4338:dbl[][])
                          n2940 = local write "Stage Moving"(TRUE ("Stage Moving")) -> ()
                          n2941 = call "move to saved stage position.vi"("Stage VISA resource name in"=w4335, "Position"=5, "Saved Stage Positions"=w4338) -> ("error out"=w4336:errorcluster)  [unwired: 1 in, 1 out]
                          n2942 = local write "Stage Control Serial Error"(w4336) -> ()
                        }
                        frame #3 {
                          w4340 = FALSE ("Stage Moving")
                          n2943 = call <vilib>:"Beep.vi"() -> ()  [unwired: 3 in, 9 out]
                          n2944 = local write "Stage Moving"(w4340) -> ()
                        }
                      }
                    }
                  }
                  n2945 = local read "Stop assembly line"() -> (w4318:bool)
                  n2946 = Not(x=w4322) -> (.not. x?=w4321:bool)
                  n2947 = node-c288() -> ()  [unwired: 1 in, 1 out]
                  n2948 = Or(x=w4321, y=w4318) -> (x .or. y?=w4320:bool)
                }
                n2949 = node-c288(w4316) -> ()  [unwired: 1 out]
              }
              frame #2 {
                n2950 = Not(x=w4346) -> (.not. x?=w4345:bool)
                n2951 = case shown="True" w4345 {
                  frame False {
                  }
                  frame True {
                    n2952 = property on="Red Laser ON" class="Bool (strict)"("Val(Sgnl)"=TRUE ("Value (Signaling)")) -> ()  [unwired: 2 in, 2 out]
                  }
                }
              }
              frame #3 {
                n2953 = node-c288() -> (w4350:T35)  [unwired: 4 in]
                n2954 = timed-loop {
                  timing: w4350 -> [_]
                  timing-out: [_] -> w4349
                  tunnel: [w4351] -> _
                  tunnel: w4348 -> [w4351]
                  stop <- "Stop assembly line" stop-if-true
                  n2955 = node-c288() -> ()  [unwired: 1 in, 1 out]
